vi "post_scan.vi"(6 "values":dbl[](array[numeric]) format="%#_8p", 8 "error in (no error)":errorcluster, 10 "config":T1={"hardware"=enum."none", "options"="", "repeats"=1, "loops"=1, "VISA"="COM7", "override_VISA"=FALSE} {"loops" min=1; "repeats" min=1}) -> (0 "error out":errorcluster)   [LabVIEW 2017]
uses:
  tools/core/var_config.ctl
  var_list.ctl
  hardware/radiant/radiant.lvlib
  tools/tools.lvlib
panel:
  # "Post-scan hardware configuration"
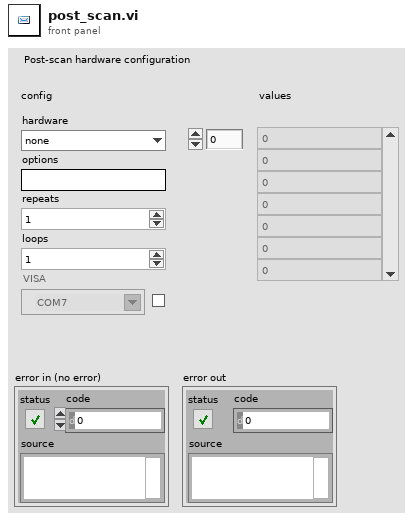
[diagram p1: front panel]
types:
  T1 = typedef "tools.lvlib/var_config.ctl" = cluster{"hardware":T2, "options":string, "repeats":i32, "loops":i32, "VISA":refnum<visa-resource-name>, "override_VISA":bool}
  T2 = typedef "var_list.ctl" = enum16{"none", "AO voltage (V)", "delay (s)", "generic", "microwaves (GHz)", "radiant (nm)", "radiant thg (nm)", "sirah (nm)", "sirah_shg (nm)", "tenma voltage (V)", "wait (s)", "wf_freq (Hz)", "wf_amp (V)", "wf_offset (V)", "wf_low_level (V)", "wf_high_level (V)", "wf_period (s)", "wf_pulse_width (s)", "wf_sample_rate (Sa/s)", "wf_multi_amp", "wf_multi_freq", "wf_arb_4chan", "WS7 setpoint (nm)"}
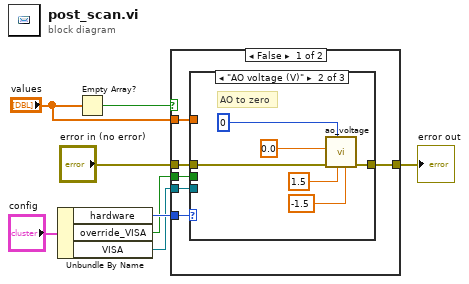
[diagram p0: block diagram]
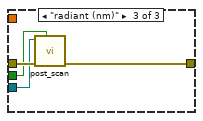
[diagram p3: hidden frame]
diagram:
  n1 = Unbundle By Name("config") -> ("hardware"=w5:T2, "override_VISA"=w3:bool, "VISA"=w4:refnum<visa-resource-name>)
  n2 = Empty Array?(array="values") -> (empty?=w2:bool)
  n3 = case shown="False" w2 {
    tunnel: "error in (no error)" -> [w14 w26]
    tunnel: [w13 w26] -> w7
    tunnel: w5 -> [w12 _]
    tunnel: w4 -> [w11 _]
    tunnel: w3 -> [w10 _]
    tunnel: "values" -> [w9 _]
    frame False {
      n4 = case shown="\"AO voltage (V)\"" w12 {
        tunnel: w14 -> [w15 w18 w25]
        tunnel: [w15 w17 w24] -> w13
        tunnel: w11 -> [_ _ w23]
        tunnel: w10 -> [_ _ w22]
        tunnel: w9 -> [_ _ _]
        frame "none", Default {
        }
        frame "AO voltage (V)" {
          # "AO to zero"
          n5 = call "ao_voltage.vi"("lower limit"=-1.5, "upper limit"=1.5, "hold (ms)"=u32 0 ("delay (ms)"), "error in"=w18, "value"=0.0) -> ("error out"=w17:errorcluster)  [unwired: 5 in, 1 out]
        }
        frame "radiant (nm)" {
          n6 = call "post_scan.vi"("override"=w22, "error in (no error)"=w25, "VISA IN"=w23) -> ("error out"=w24:errorcluster)  [unwired: 8 in]
        }
      }
    }
    frame True {
    }
  }
  "error out" <- w7
